vi "Write to File.vi"(8 "error in (no error)":errorcluster, 10 "INI Ref":T1, 11 "Step in":refnum<class "Step.lvclass">) -> (0 "error out":errorcluster, 2 "INI Ref out":T1, 3 "Step out":refnum<class "Step.lvclass">)   [LabVIEW 2020, in "MacroAssert.lvlib" / "Step.lvclass"]
uses:
  Step.lvclass
  Step.lvclass/Step.ctl
  MacroAssert.lvlib
  <vilib>/Utility/config.llb/NI_LVConfig.lvlib
  <vilib>/Utility/config.llb/Write Key (String).vi
  <vilib>/Utility/config.llb/Write Key (I32).vi
  <vilib>/Utility/config.llb/Config Data RefNum.ctl
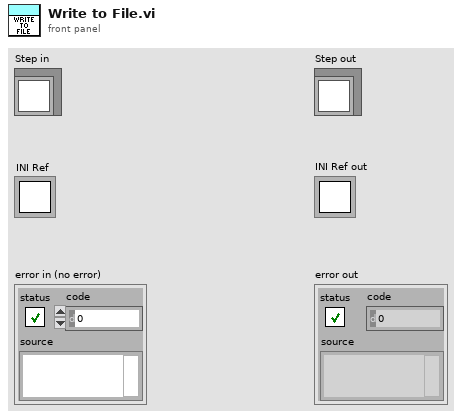
[diagram p1: front panel]
types:
  T1 = typedef "NI_LVConfig.lvlib/Config Data RefNum.ctl" = refnum<k1>
  T2 = typedef "MacroAssert.lvlib/Step Type V3.ctl" = enum16{"Mouse Action", "Keyboard Action", "Window Action", "Timing Action", "Boolean Assertion", "Numeric Assertion", "String Assertion", "Image Assertion"}
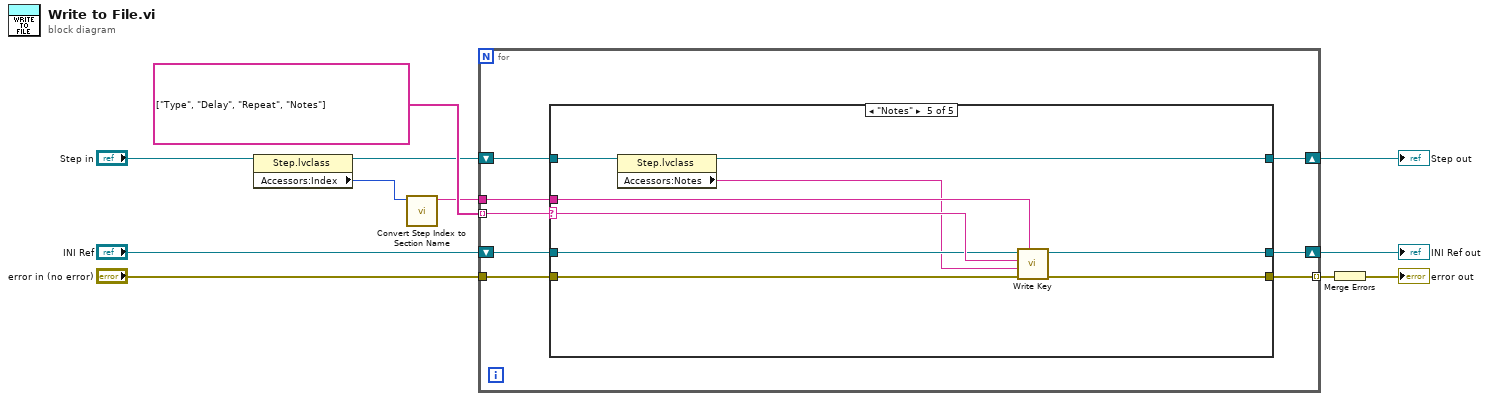
[diagram p0: block diagram]
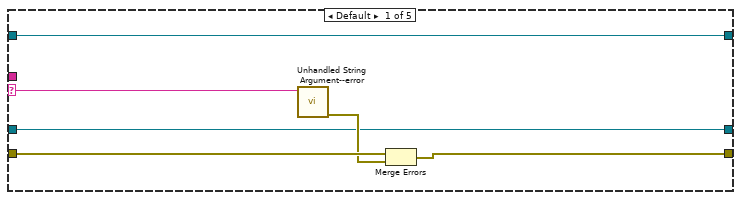
[diagram p2: hidden frame]
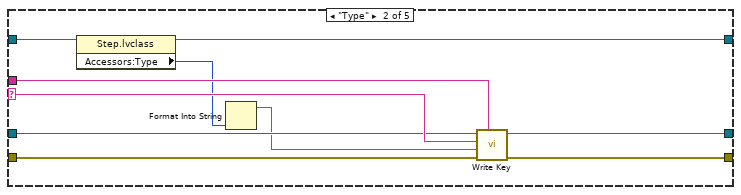
[diagram p3: hidden frame]
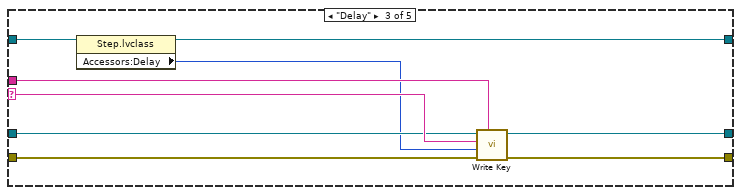
[diagram p4: hidden frame]
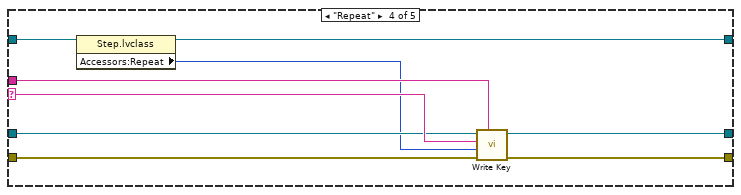
[diagram p5: hidden frame]
diagram:
  n1 = property class="Step.lvclass"(reference="Step in") -> (reference out=w8:refnum<class "Step.lvclass">, "Accessors:Index"=w11:i32)  [unwired: 1 in, 1 out]
  n2 = call "Convert Step Index to Section Name.vi"("Step Index"=w11) -> ("Section Name"=w7:string)  [unwired: 10 in]
  n3 = for {
    tunnel: string[] ["Type", "Delay", "Repeat", "Notes"] -> [w19] mode=indexing
    tunnel: "error in (no error)" -> [w18]
    tunnel: w7 -> [w17]
    shift-right: [w15] -> w1
    shift-left: w8 -> [w16]
    tunnel: [w14] -> w9 mode=indexing
    shift-right: [w12] -> w2
    shift-left: "INI Ref" -> [w13]
    n4 = case shown="\"Notes\"" w19 {
      selector: w19 -> [w22 w33 w42 w51 w60]
      tunnel: w18 -> [w24 w35 w44 w53 w62]
      tunnel: w17 -> [_ w34 w43 w52 w61]
      tunnel: w16 -> [w25 w31 w40 w49 w58]
      tunnel: [w25 w26 w37 w46 w55] -> w15
      tunnel: [w21 w30 w39 w48 w57] -> w14
      tunnel: w13 -> [w20 w32 w41 w50 w59]
      tunnel: [w20 w29 w38 w47 w56] -> w12
      frame Default {
        n5 = call "Unhandled String Argument--error.vi"("Argument"=w22) -> ("error out"=w23:errorcluster)  [unwired: 10 in]
        n6 = Merge Errors(w24, w23) -> (w21:errorcluster)
      }
      frame "Type" {
        n7 = property class="Step.lvclass"(reference=w31) -> (reference out=w26:refnum<class "Step.lvclass">, "Accessors:Type"=w28:T2)  [unwired: 1 in, 1 out]
        n8 = Format Into String(w28) -> (resulting string=w27:string)  [unwired: 3 in, 1 out]
        n9 = call-poly <vilib>:"Write Key.vi"("section"=w34, "error in (no error)"=w35, "value"=w27, "key"=w33, "refnum"=w32) -> ("error out"=w30:errorcluster, "refnum out"=w29:T1)  [unwired: 4 in, 1 out]
      }
      frame "Delay" {
        n10 = property class="Step.lvclass"(reference=w40) -> (reference out=w37:refnum<class "Step.lvclass">, "Accessors:Delay"=w36:i32)  [unwired: 1 in, 1 out]
        n11 = call-poly <vilib>:"Write Key.vi"("section"=w43, "error in (no error)"=w44, "value"=w36, "key"=w42, "refnum"=w41) -> ("error out"=w39:errorcluster, "refnum out"=w38:T1)  [unwired: 4 in, 1 out]
      }
      frame "Repeat" {
        n12 = property class="Step.lvclass"(reference=w49) -> (reference out=w46:refnum<class "Step.lvclass">, "Accessors:Repeat"=w45:i32)  [unwired: 1 in, 1 out]
        n13 = call-poly <vilib>:"Write Key.vi"("section"=w52, "error in (no error)"=w53, "value"=w45, "key"=w51, "refnum"=w50) -> ("error out"=w48:errorcluster, "refnum out"=w47:T1)  [unwired: 4 in, 1 out]
      }
      frame "Notes" {
        n14 = property class="Step.lvclass"(reference=w58) -> (reference out=w55:refnum<class "Step.lvclass">, "Accessors:Notes"=w54:string)  [unwired: 1 in, 1 out]
        n15 = call-poly <vilib>:"Write Key.vi"("section"=w61, "error in (no error)"=w62, "value"=w54, "key"=w60, "refnum"=w59) -> ("error out"=w57:errorcluster, "refnum out"=w56:T1)  [unwired: 4 in, 1 out]
      }
    }
  }
  "Step out" <- w1
  "INI Ref out" <- w2
  n16 = Merge Errors(w9) -> (→"error out":errorcluster)
